vi "2D-U16_SubpixelShift.vi"(7 "Shift in y":bool=TRUE, 10 "Shift":dbl=0.5, 11 "U16-Array":u16[][](array[numeric])=[[1, 4, 7, 9], [2, 5, 8, 10], [3, 6, 9, 11], [4, 7, 10, 12], [5, 8, 11, 13], [6, 9, 12, 14]]) -> (3 "U16-Array result":u16[][](array[numeric])=[[1, 4, 7, 9], [2, 4, 8, 10], [2, 6, 8, 10], [4, 6, 10, 12], [4, 8, 10, 12], [6, 8, 12, 14]])   [LabVIEW 2011]
panel:
  # "< x-shift in this direction, 2. Dimmension"
  # "I"
  # "<>"
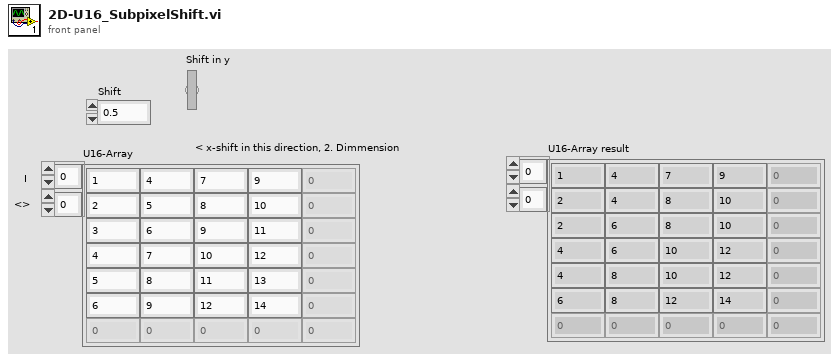
[diagram p1: front panel]
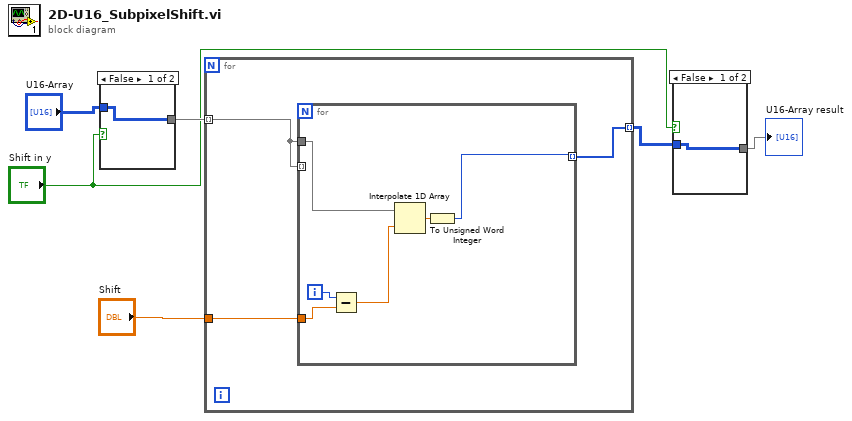
[diagram p0: block diagram]
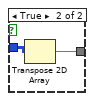
[diagram p2: hidden frame]
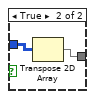
[diagram p3: hidden frame]
diagram:
  n1 = case shown="False" "Shift in y" {
    tunnel: "U16-Array" -> [w7 w9]
    tunnel: [w7 w8] -> w4
    frame False {
    }
    frame True {
      n2 = Transpose 2D Array(2D array=w9) -> (transposed array=w8:u16[][])
    }
  }
  n3 = for {
    tunnel: w4 -> [w10] mode=indexing
    tunnel: "Shift" -> [w12]
    tunnel: [w11] -> w2 mode=indexing
    n4 = for {
      tunnel: w10 -> [w18]
      tunnel: w12 -> [w14]
      tunnel: [w16] -> w11 mode=indexing
      tunnel: w10 -> [_] mode=indexing
      i -> [w15]
      n5 = Subtract(x=w15, y=w14) -> (x-y=w13:dbl)
      n6 = Interpolate 1D Array(1:w13, 2:w18) -> (0:w17:dbl)
      n7 = To Unsigned Word Integer(number=w17) -> (unsigned 16bit integer=w16:u16)
    }
  }
  n8 = case shown="False" "Shift in y" {
    tunnel: w2 -> [w19 w21]
    tunnel: [w19 w20] -> w1
    frame False {
    }
    frame True {
      n9 = Transpose 2D Array(2D array=w21) -> (transposed array=w20:u16[][])
    }
  }
  "U16-Array result" <- w1
